vi "K8005 test.vi"() -> ()   [LabVIEW 2024]
panel:
  in  "stop":bool
  in  "Boolean":bool
  out "Thermometer":dbl(slide) scale=0.0..100.0
  in  "Knob":dbl(knob) scale=0.0..10.0
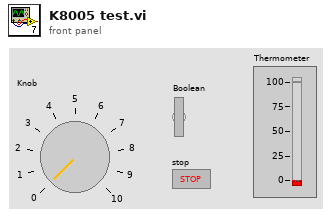
[diagram p1: front panel]
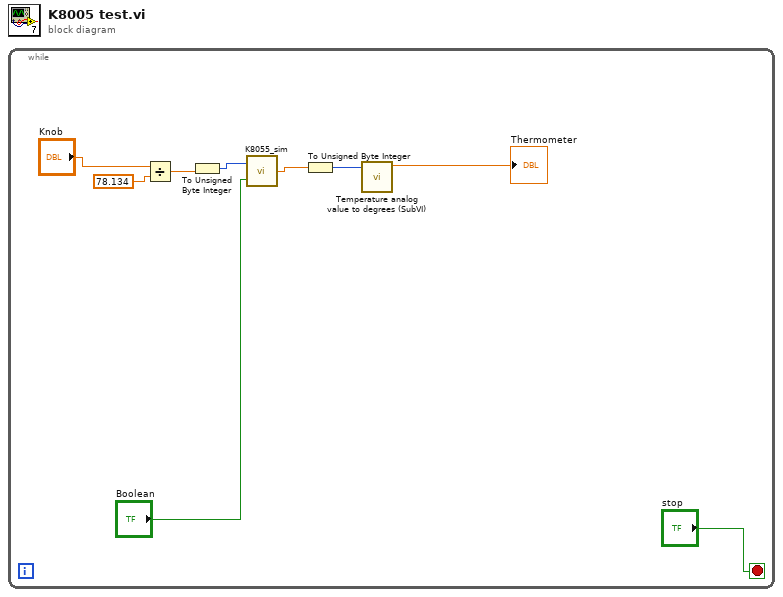
[diagram p0: block diagram]
diagram:
  n1 = while {
    stop <- "stop" stop-if-true
    n2 = Divide(x="Knob", y=78.134) -> (x/y=w5:dbl)
    n3 = To Unsigned Byte Integer(number=w5) -> (unsigned 8bit integer=w3:u8)
    n4 = call "K8055_sim.vi"("Hardware"="Boolean", "Fan Speed"=w3) -> ("Read temp"=w2:dbl)
    n5 = To Unsigned Byte Integer(number=w2) -> (unsigned 8bit integer=w4:u8)
    n6 = call "Temperature analog value to degrees (SubVI).vi"("Temperature Analog Value"=w4) -> ("Temperature (C)"=→"Thermometer":dbl)  [unwired: 10 in]
  }
